vi "MVE Create N Variables.vi"(11 "Path":string) -> (0 "error out":errorcluster, 3 "cancelled":bool)   [LabVIEW 2016]
uses:
  <vilib>/variable/NI_Variable.lvlib
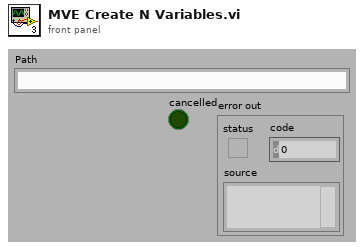
[diagram p1: front panel]
types:
  T1 = typedef "NI_Variable.lvlib/variable.ctl" = cluster{"Name":string, "TypeDesc":T2, "Type":string, "Typedefs":string, "Attribs":T3, "FeaturePacks":string[]}
  T2 = typedef "NI_Variable.lvlib/Type Descriptor.ctl" = cluster{"Variant":variant}
  T3 = typedef "NI_Variable.lvlib/Attribs.ctl" = cluster{"Attrib":string, "Value":string}[]
  T4 = typedef "SCT Variable.ctl" = cluster{"Name":string, "TypeDesc":T2, "Type":string, "typedefs":string, "Attribs":T3, "FeaturePacks":string[], "Source":string}
  T5 = typedef "SCT Default Types.ctl" = cluster{"names":string[], "TDs":T2[]}
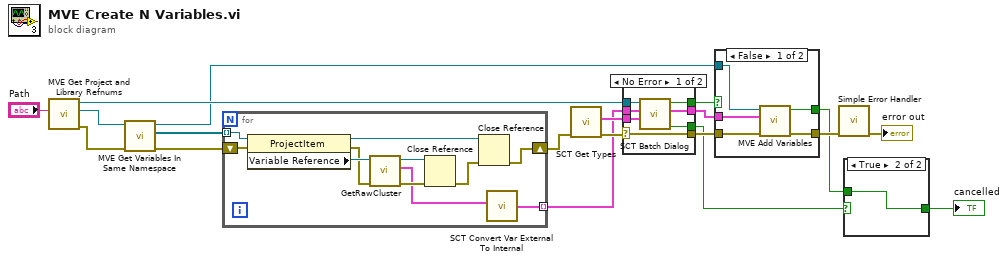
[diagram p0: block diagram]
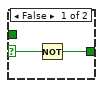
[diagram p2: hidden frame]
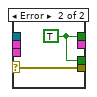
[diagram p3: hidden frame]
diagram:
  n1 = call <resource>:"MVE Get Project and Library Refnums.vi"("Full Path"="Path") -> ("error out"=w3:errorcluster, "ProjectItem Refnum"=w10:refnum<vi>, "Project Refnum"=w19:refnum<vi>)  [unwired: 8 in]
  n2 = call <resource>:"MVE Get Variables In Same Namespace.vi"("error in (no error)"=w3, "ProjectItem Refnum"=w10) -> ("error out"=w2:errorcluster, "Variable Children"=w1:refnum<vi>[], "dup ProjectItem Refnum"=w9:refnum<vi>)  [unwired: 7 in]
  n3 = for {
    tunnel: [w25] -> w7 mode=indexing
    shift-right: [w22] -> w8
    shift-left: w2 -> [w29]
    tunnel: w1 -> [w20] mode=indexing
    n4 = property class="ProjectItem"(reference=w20, error in=w29) -> (reference out=w23:refnum<vi>, error out=w28:errorcluster, "Variable Reference"=w30:refnum<vi>)
    n5 = call <vilib>:"GetRawCluster.vi"("error in (no error)"=w28, "Variable Reference in"=w30) -> ("error out"=w27:errorcluster, "Variable"=w26:T1, "Variable Reference out"=w21:refnum<vi>)  [unwired: 7 out]
    n6 = Close Reference(reference=w21, error in (no error)=w27) -> (error out=w24:errorcluster)
    n7 = Close Reference(reference=w23, error in (no error)=w24) -> (error out=w22:errorcluster)
    n8 = call <resource>:"SCT Convert Var External To Internal.vi"("External Var"=w26) -> ("Internal Var"=w25:T4)  [unwired: 1 in, 4 out]
  }
  n9 = call <resource>:"SCT Get Types.vi"("error in"=w8) -> ("error out"=w15:errorcluster, "default types"=w17:T5)  [unwired: 8 in, 1 out]
  n10 = case shown="No Error" w15 {
    selector: w15 -> [w33 w39]
    tunnel: w19 -> [w37 _]
    tunnel: w17 -> [w36 _]
    tunnel: [w35 w38] -> w11
    tunnel: [w34 _] -> w16
    tunnel: [w33 w39] -> w14
    tunnel: w7 -> [w31 _]
    tunnel: [w32 w38] -> w6
    frame No Error {
      n11 = call <resource>:"SCT Batch Dialog.vi"("default types"=w36, "VariablesIn"=w31, "Project Refnum"=w37) -> ("ShowMVE?"=w32:bool, "VariablesOut"=w34:T4[], "Cancelled?"=w35:bool)  [unwired: 5 in, 1 out]
    }
    frame Error {
      w38 = TRUE ("Cancelled?")
    }
  }
  n12 = case shown="False" w11 {
    selector: w11 -> [_ w45]
    tunnel: w16 -> [w40 _]
    tunnel: w14 -> [w44 w46]
    tunnel: [w42 w46] -> w13
    tunnel: w9 -> [w43 _]
    tunnel: [w41 w45] -> w4
    frame False {
      n13 = call <resource>:"MVE Add Variables.vi"("error in (no error)"=w44, "variables"=w40, "ProjectItem Refnum"=w43) -> ("error out"=w42:errorcluster, "cancelled"=w41:bool)  [unwired: 7 in]
    }
    frame True {
    }
  }
  n14 = call <vilib>:"Simple Error Handler.vi"("error in (no error)"=w13) -> ("error out"=→"error out":errorcluster)  [unwired: 4 in, 4 out]
  n15 = case shown="True" w6 {
    selector: w6 -> [w48 _]
    tunnel: [w47 w49] -> w5
    tunnel: w4 -> [_ w49]
    frame False {
      n16 = Not(x=w48) -> (.not. x?=w47:bool)
    }
    frame True {
    }
  }
  "cancelled" <- w5
